vi "Frequency Offset Compensation.vi"(5 "use static frequency shift":bool=TRUE, 7 "static frequency shift":fxp<+/-,48,0>, 8 "estimated frequency shift valid":bool=TRUE, 9 "estimated frequency shift":fxp<+/-,48,0>, 10 "sample in valid":bool=TRUE, 11 "channels in":T1) -> (0 "compensated CFO":fxp<+/-,48,0>, 1 "output valid":bool=TRUE, 2 "channels out":T1)   [LabVIEW 2020]
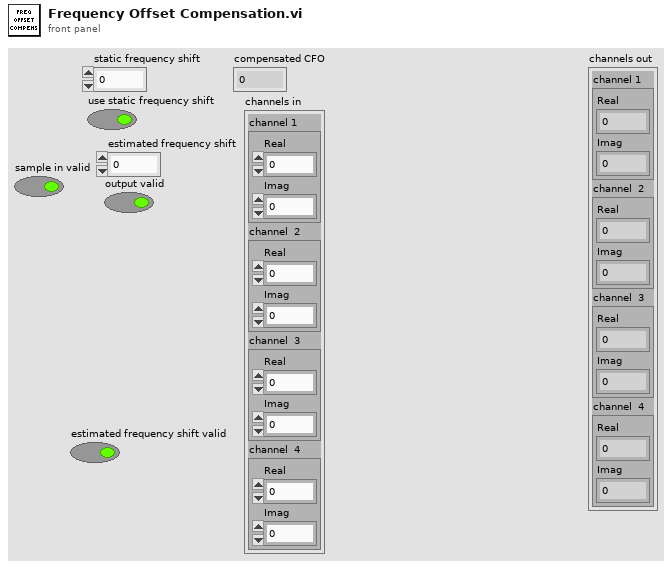
[diagram p1: front panel]
types:
  T1 = cluster{"channel 1 ":cluster{"Real":fxp<+/-,16,3>, "Imag":fxp<+/-,16,3>}, "channel  2":cluster{"Real":fxp<+/-,16,3>, "Imag":fxp<+/-,16,3>}, "channel  3":cluster{"Real":fxp<+/-,16,3>, "Imag":fxp<+/-,16,3>}, "channel  4":cluster{"Real":fxp<+/-,16,3>, "Imag":fxp<+/-,16,3>}}
  T2 = cluster{"sample in valid":bool, "static frequency shift":fxp<+/-,48,0>, "use static frequency shift":bool, "estimated frequency shift":fxp<+/-,48,0>, "estimated frequency shift valid":bool}
  T3 = cluster{"Real":fxp<+/-,16,3>, "Imag":fxp<+/-,16,3>}
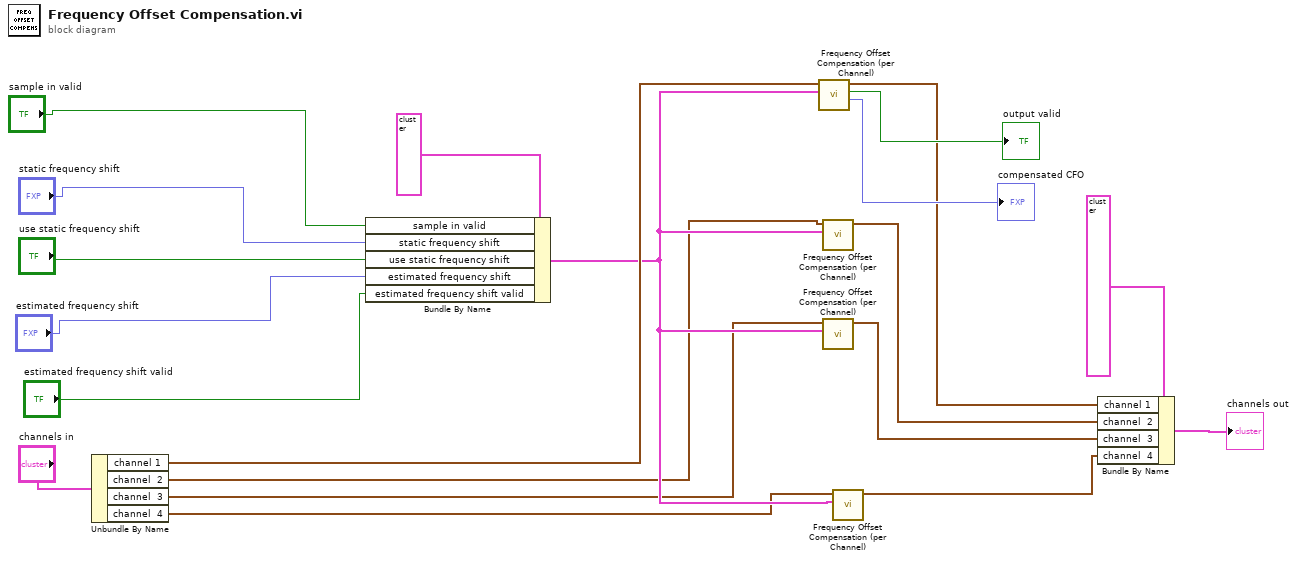
[diagram p0: block diagram]
diagram:
  n1 = Unbundle By Name("channels in") -> ("channel 1"=w11:T3, "channel  2"=w9:T3, "channel  3"=w8:T3, "channel  4"=w7:T3)
  n2 = Bundle By Name(cluster=T2 {"sample in valid"=FALSE, "static frequency shift"=0.0, "use static frequency shift"=FALSE, "estimated frequency shift"=0.0, "estimated frequency shift valid"=FALSE}, "sample in valid"="sample in valid", "static frequency shift"="static frequency shift", "use static frequency shift"="use static frequency shift", "estimated frequency shift"="estimated frequency shift", "estimated frequency shift valid"="estimated frequency shift valid") -> (w10:T2)
  n3 = call "Frequency Offset Compensation (per Channel).vi"("params"=w10, "sample in"=w11) -> ("static frequency shift out"=→"compensated CFO":fxp<+/-,48,0>, "output valid"=→"output valid":bool, "sample out"=w2:T3)  [unwired: 7 in]
  n4 = call "Frequency Offset Compensation (per Channel).vi"("params"=w10, "sample in"=w9) -> ("sample out"=w3:T3)  [unwired: 7 in, 2 out]
  n5 = call "Frequency Offset Compensation (per Channel).vi"("params"=w10, "sample in"=w8) -> ("sample out"=w4:T3)  [unwired: 7 in, 2 out]
  n6 = call "Frequency Offset Compensation (per Channel).vi"("params"=w10, "sample in"=w7) -> ("sample out"=w5:T3)  [unwired: 7 in, 2 out]
  n7 = Bundle By Name(cluster=T1 {"channel 1 "={"Real"=0.0, "Imag"=0.0}, "channel  2"={"Real"=0.0, "Imag"=0.0}, "channel  3"={"Real"=0.0, "Imag"=0.0}, "channel  4"={"Real"=0.0, "Imag"=0.0}} ("channels in"), "channel 1"=w2, "channel  2"=w3, "channel  3"=w4, "channel  4"=w5) -> (→"channels out":T1)
